vi "Set Paths.vi"(7 "Measurement specfic paths":T1=enum."Harmonics", 8 "error in (no error)":errorcluster, 11 "Manual Switch in":refnum<class "Manual Switch.lvclass">) -> (0 "error out":errorcluster, 3 "Manual Switch out":refnum<class "Manual Switch.lvclass">)   [LabVIEW 2020, in "Manual Switch.lvclass"]
uses:
  Manual Switch.lvclass
  Path Control/Measurements Specific Paths.ctl
  Path Control/PathControl.lvclass
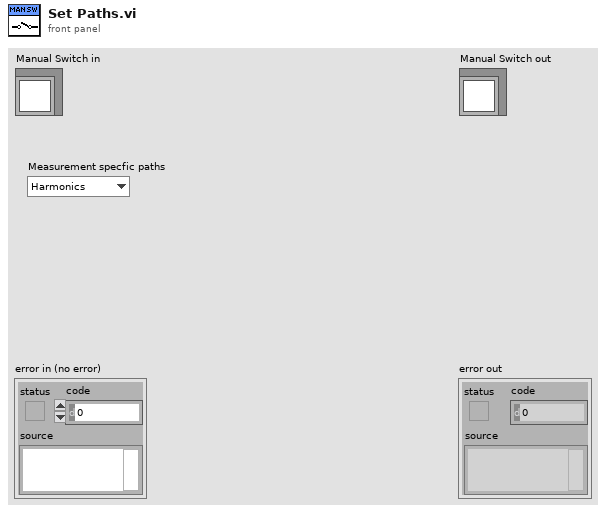
[diagram p1: front panel]
types:
  T1 = typedef "PathControl.lvclass/Measurements Specific Paths.ctl" = enum16{"No calibration", "Harmonics", "IMD", "S Parameter", "AM-AM", "MCCW-ACLR", "DC", "LCR", "Power Meter GUI", "RF Power"}
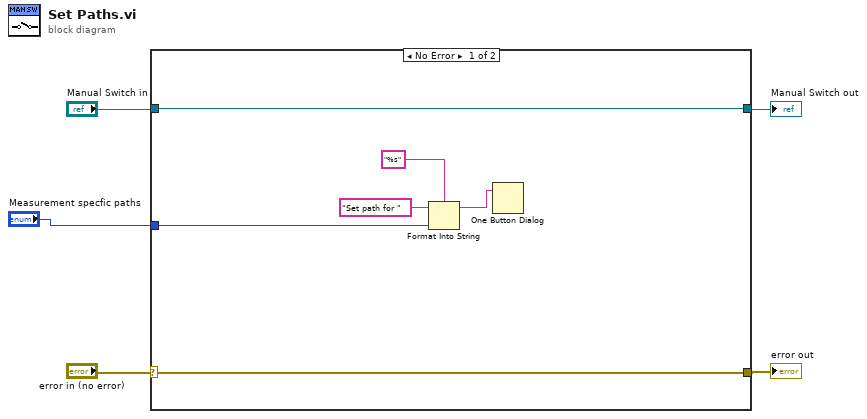
[diagram p0: block diagram]
diagram:
  n1 = case shown="No Error" "error in (no error)" {
    selector: "error in (no error)" -> [w10 w13]
    tunnel: [w10 w13] -> w5
    tunnel: [w11 w12] -> w3
    tunnel: "Manual Switch in" -> [w11 w12]
    tunnel: "Measurement specfic paths" -> [w6 _]
    frame No Error {
      n2 = Format Into String(format string="%s", initial string="Set path for ", w6) -> (resulting string=w7:string)  [unwired: 1 in, 1 out]
      n3 = One Button Dialog(message=w7) -> ()  [unwired: 1 in, 1 out]
    }
    frame Error {
    }
  }
  "error out" <- w5
  "Manual Switch out" <- w3
